vi "fmt_formatSingleCell.vi"(4 "style":string, 5 "format string":string, 6 "index":i32, 7 "column":string, 8 "error in (no error)":errorcluster, 9 "data":T1, 10 "row":i32, 11 "Format buffer":u8[](array[numeric])) -> (0 "error out":errorcluster, 1 "Formatted data length":i32, 2 "Buffer size":i32, 3 "Formatted buffer":u8[](array[numeric]))   [LabVIEW 2017, in "NI_ExcelFile.lvlib"]
uses:
  <vilib>/express/express shared/NI_ExcelFile/NI_ExcelFile.lvlib
  <vilib>/express/express shared/NI_ExcelFile/Ctrls/data_AllTypeData.ctl
  <vilib>/express/express shared/NI_ExcelFile/Ctrls/DataType.ctl
  <vilib>/express/express shared/NI_ExcelFile/SubVIs/fmt_escapeXML.vi
  <vilib>/express/express shared/NI_ExcelFile/SubVIs/fmt_getUTF-8Text.vi
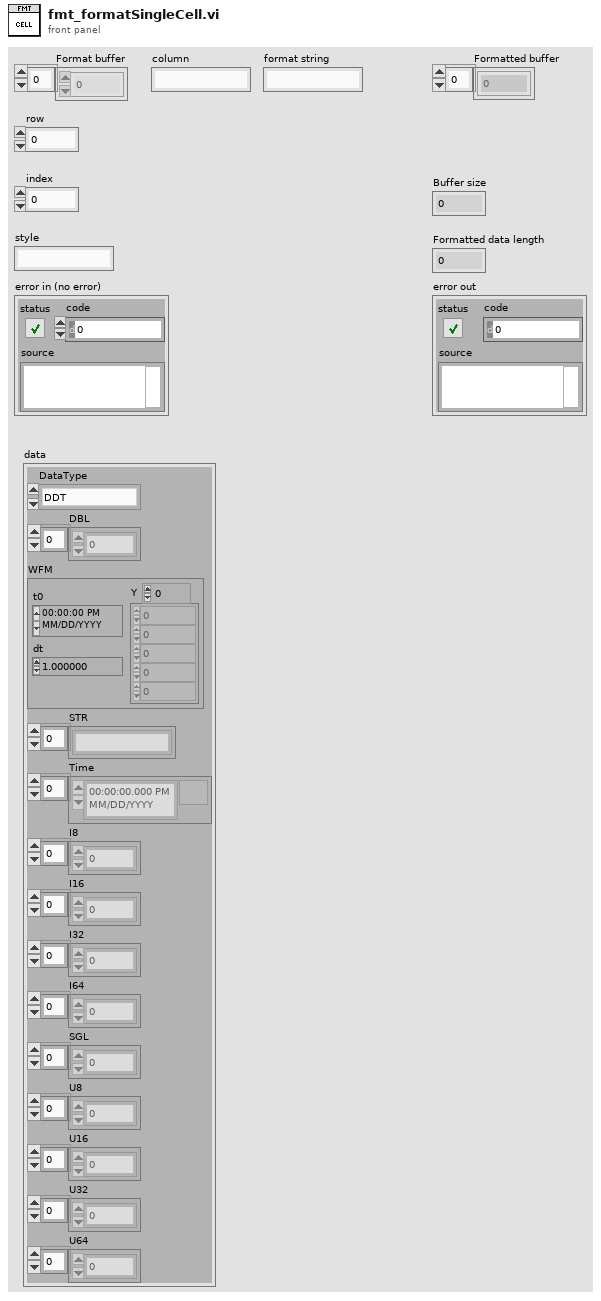
[diagram p1: front panel]
types:
  T1 = typedef "NI_ExcelFile.lvlib/data_AllTypeData.ctl" = cluster{"DataType":T2, "DBL":dbl[], "WFM":waveform(dbl), "STR":string[], "Time":timestamp[], "I8":i8[], "I16":i16[], "I32":i32[], "I64":i64[], "SGL":sgl[], "U8":u8[], "U16":u16[], "U32":u32[], "U64":u64[]}
  T2 = typedef "NI_ExcelFile.lvlib/DataType.ctl" = enum16{"DDT", "WFM", "Array of STR", "Array of DBL", "Array of I8", "Array of I16", "Array of I32", "Array of I64", "Array of SGL", "Array of U8", "Array of U16", "Array of U32", "Array of U64", "Array of Time"}
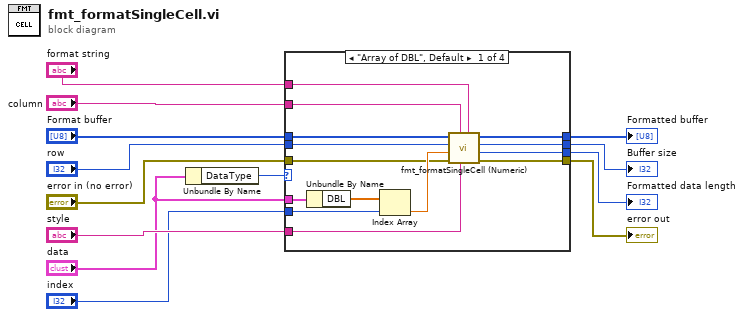
[diagram p0: block diagram]
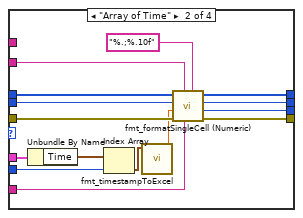
[diagram p2: hidden frame]
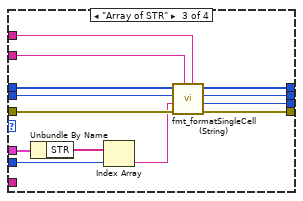
[diagram p3: hidden frame]
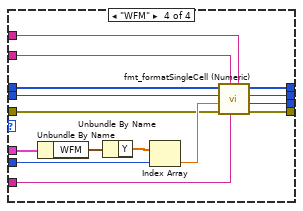
[diagram p4: hidden frame]
diagram:
  n1 = Unbundle By Name("data") -> ("DataType"=w1:T2)
  n2 = case shown="\"Array of DBL\", Default" w1 {
    tunnel: "data" -> [w27 w42 w55 w59]
    tunnel: "index" -> [w25 w40 w53 w57]
    tunnel: "column" -> [w23 w39 w52 w63]
    tunnel: "format string" -> [w22 _ w51 w64]
    tunnel: "Format buffer" -> [w21 w38 w50 w62]
    tunnel: "row" -> [w20 w37 w49 w61]
    tunnel: "error in (no error)" -> [w19 w36 w48 w60]
    tunnel: "style" -> [w18 w35 _ w56]
    tunnel: [w17 w34 w47 w68] -> w10
    tunnel: [w16 w33 w46 w67] -> w9
    tunnel: [w15 w32 w45 w66] -> w8
    tunnel: [w14 w31 w44 w65] -> w7
    frame "Array of DBL", Default {
      n3 = Unbundle By Name(w27) -> ("DBL"=w26:dbl[])
      n4 = Index Array(array=w26, index=w25) -> (element=w24:dbl)
      n5 = call <vilib>:"fmt_formatSingleCell (Numeric).vi"("format string"=w22, "style index"=w18, "Column"=w23, "error in"=w19, "Value"=w24, "Row"=w20, "Format buffer"=w21) -> ("error out"=w17:errorcluster, "Formatted data length"=w16:i32, "Buffer size"=w15:i32, "Formatted buffer"=w14:u8[])  [unwired: 1 in]
    }
    frame "Array of Time" {
      n6 = Unbundle By Name(w42) -> ("Time"=w41:timestamp[])
      n7 = Index Array(array=w41, index=w40) -> (element=w30:timestamp)
      n8 = call <vilib>:"fmt_timestampToExcel.vi"("timestamp"=w30) -> ("Excel timestamp"=w29:dbl)  [unwired: 10 in]
      n9 = call <vilib>:"fmt_formatSingleCell (Numeric).vi"("format string"="%.;%.10f", "style index"=w35, "Column"=w39, "error in"=w36, "Value"=w29, "Row"=w37, "Format buffer"=w38) -> ("error out"=w34:errorcluster, "Formatted data length"=w33:i32, "Buffer size"=w32:i32, "Formatted buffer"=w31:u8[])  [unwired: 1 in]
    }
    frame "Array of STR" {
      n10 = Unbundle By Name(w55) -> ("STR"=w54:string[])
      n11 = Index Array(array=w54, index=w53) -> (element=w43:string)
      n12 = call <vilib>:"fmt_formatSingleCell (String).vi"("format string"=w51, "column"=w52, "error in"=w48, "data"=w43, "row"=w49, "format buffer"=w50) -> ("error out"=w47:errorcluster, "formatted value length"=w46:i32, "buffer size"=w45:i32, "formatted buffer"=w44:u8[])  [unwired: 2 in]
    }
    frame "WFM" {
      n13 = Unbundle By Name(w59) -> ("WFM"=w69:waveform(dbl))
      n14 = Unbundle By Name(w69) -> ("Y"=w58:dbl[])
      n15 = Index Array(array=w58, index=w57) -> (element=w70:dbl)
      n16 = call <vilib>:"fmt_formatSingleCell (Numeric).vi"("format string"=w64, "style index"=w56, "Column"=w63, "error in"=w60, "Value"=w70, "Row"=w61, "Format buffer"=w62) -> ("error out"=w68:errorcluster, "Formatted data length"=w67:i32, "Buffer size"=w66:i32, "Formatted buffer"=w65:u8[])  [unwired: 1 in]
    }
  }
  "error out" <- w10
  "Formatted data length" <- w9
  "Buffer size" <- w8
  "Formatted buffer" <- w7
